vi "Configure Output Enabled.vi"(8 "error in (no error)":errorcluster, 9 "Output Enabled (F: Off)":bool, 11 "VISA resource name":refnum<visa-resource-name>) -> (0 "error out":errorcluster, 3 "VISA resource name out":refnum<visa-resource-name>)   [LabVIEW 2013]
doc: "Configures whether the signal that the power supply produces on a channel appears at the output connector."
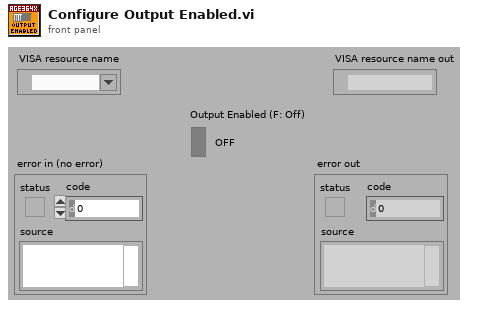
[diagram p1: front panel]
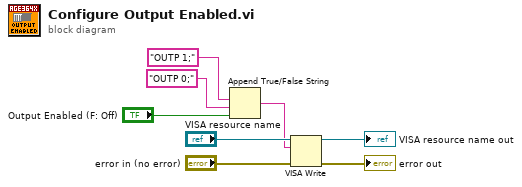
[diagram p0: block diagram]
diagram:
  n1 = Append True/False String(1:"Output Enabled (F: Off)", 2:"OUTP 0;" ("false string"), 3:"OUTP 1;" ("true string")) -> (0:w1:string)  [unwired: 1 in]
  n2 = VISA Write(VISA resource name="VISA resource name", write buffer=w1, error in (no error)="error in (no error)") -> (VISA resource name out=→"VISA resource name out":refnum<visa-resource-name>, error out=→"error out":errorcluster)  [unwired: 1 out]
